vi "spectralDemo.vi"() -> ()   [LabVIEW 2024]
uses:
  <vilib>/express/express analysis/Spectral/Block/exnSpectralBlock spectral measurements RMS poly.vi
  <vilib>/express/express analysis/Spectral/Block/exnSpectralBlock spectral measurements RMS DDT.vi
  <vilib>/express/express analysis/Spectral/XNode/ExpressSpectralMeasurementsBlockNode.xnode
panel:
  out "Waveform Graph":dynamicdata(graph)
  out "Waveform Graph 2":dynamicdata(graph)
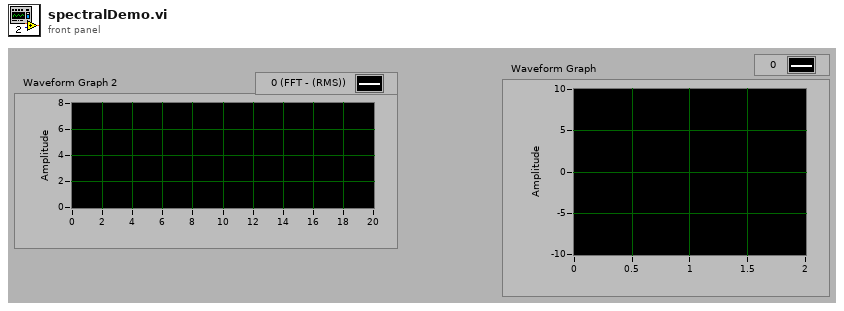
[diagram p1: front panel]
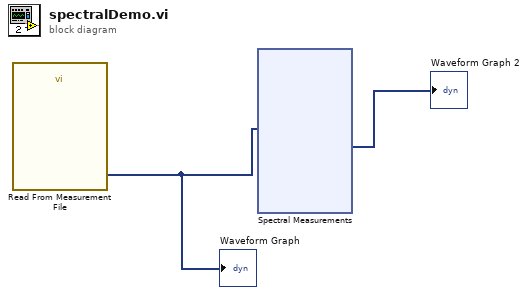
[diagram p0: block diagram]
diagram:
  n1 = call "Read From Measurement File"() -> ("Signals"=w1:dynamicdata)  [unwired: 6 in, 5 out]
  "Waveform Graph" <- w1
  n2 = xnode "Spectral Measurements"("Signals"=w1) -> ("FFT - (RMS)"=→"Waveform Graph 2":dynamicdata)  [unwired: 2 in, 3 out]
